vi "Control - Generic - VVA Host.vi"() -> ()   [LabVIEW 2015, in "ECS-Host.lvlib"]
uses:
  ECS-Host.lvlib
  <vilib>/addons/Software Calibration Management/XControls/TBL2D.xctl
panel:
  in  "Cam2Adv_ManE":bool
  in  "Cam2Adv_Man":sgl caption="[DBTDC]"
  out "Cam2Adv_Des":sgl caption="[DBTDC]"
  out "Cam2Adv_TblOut":sgl caption="[DBTDC]"
  in  "Cam2Adv_Tbl":cluster{"X":sgl[], "Y":sgl[], "Z":sgl[][]}(xcontrol) caption="[DBTDC]"
  in  "Cam1Adv_ManE":bool
  in  "Cam1Adv_Man":sgl caption="[DBTDC]"
  out "Cam1Adv_Des":sgl caption="[DBTDC]"
  out "Cam1Adv_TblOut":sgl caption="[DBTDC]"
  in  "Cam1Adv_Tbl":cluster{"X":sgl[], "Y":sgl[], "Z":sgl[][]}(xcontrol) caption="[DBTDC]"
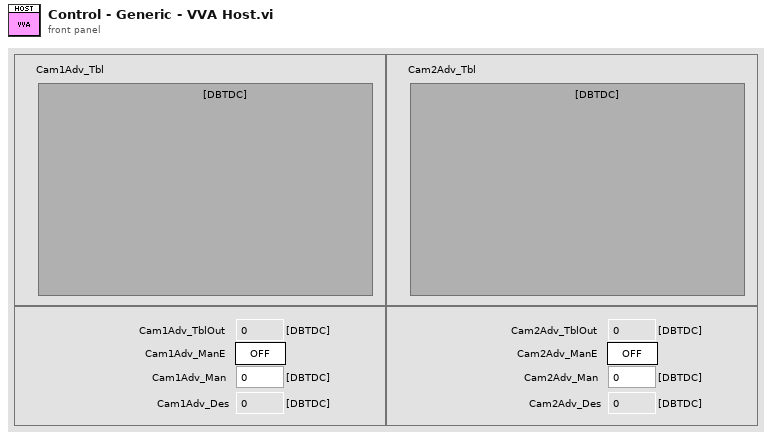
[diagram p1: front panel]
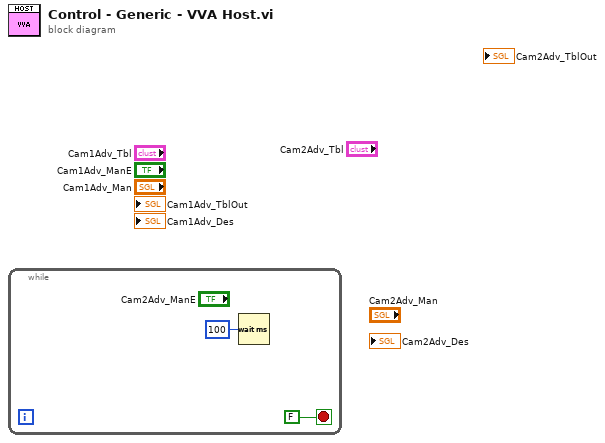
[diagram p0: block diagram]
diagram:
  n1 = while {
    stop <- FALSE stop-if-true
    n2 = Wait (ms)(milliseconds to wait=u32 100) -> ()  [unwired: 1 out]
  }
